vi "Evaluate Log Packet.vi"(10 "Log Packet":T1, 11 "Log Sink in":refnum<class "Log Sink.lvclass">) -> (1 "Log?":bool, 2 "Log Packet Out":T1, 3 "Log Sink out":refnum<class "Log Sink.lvclass">)   [LabVIEW 2019, in "Composed Log.lvlib" / "Log Sink.lvclass"]
uses:
  <vilib>/gpm_packages/@cs/event-logger/Source/Composed Log/Log Sink/Log Sink.lvclass
  <vilib>/gpm_packages/@cs/event-logger/Source/Composed Log/Types/Log Packet.ctl
  <vilib>/gpm_packages/@cs/event-logger/Source/Composed Log/Types/Log Level.ctl
  <vilib>/gpm_packages/@cs/event-logger/Source/Composed Log/Log Sink/Log Sink.lvclass/Log Sink.ctl
  <vilib>/gpm_packages/@cs/event-logger/Source/Composed Log/ILogFilter/ILogFilter.lvclass
  <vilib>/gpm_packages/@cs/event-logger/Source/Composed Log/Composed Log.lvlib
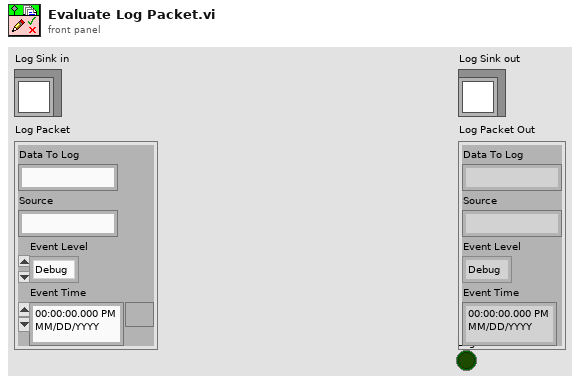
[diagram p1: front panel]
types:
  T1 = typedef "Composed Log.lvlib/Log Packet.ctl" = cluster{"Data To Log":string, "Source":string, "Event Level":T2, "Event Time":timestamp}
  T2 = typedef "Composed Log.lvlib/Log Level.ctl" = enum16{"Debug", "Info", "Warning", "Error", "Critical"}
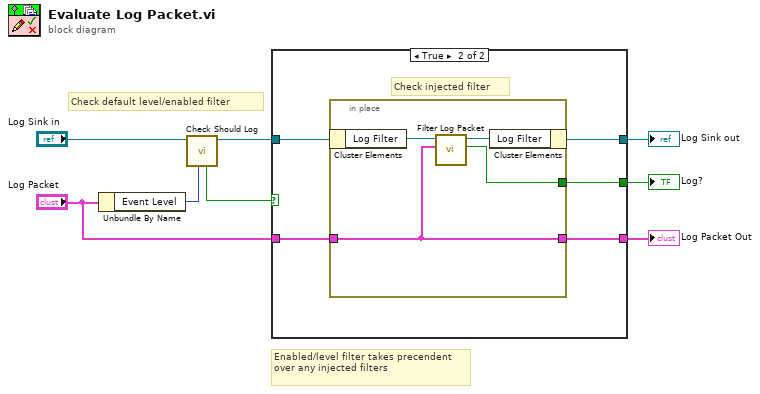
[diagram p0: block diagram]
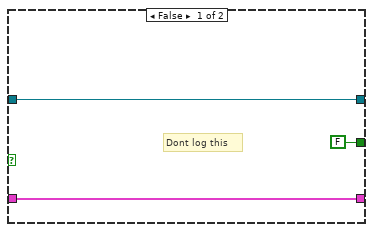
[diagram p2: hidden frame]
diagram:
  # "Enabled/level filter takes precendent over any injected filters"
  # "Check default level/enabled filter"
  n1 = Unbundle By Name("Log Packet") -> ("Event Level"=w7:T2)
  n2 = call <vilib>:"Check Should Log.vi"("LogLevel"=w7, "Log Sink in"="Log Sink in") -> ("Log Sink out"=w6:refnum<class "Log Sink.lvclass">, "Log?"=w5:bool)  [unwired: 8 in]
  n3 = case shown="True" w5 {
    tunnel: w6 -> [w11 w15]
    tunnel: "Log Packet" -> [w9 w16]
    tunnel: [w11 w14] -> w3
    tunnel: [FALSE ("Log?") w13] -> w2
    tunnel: [w9 w12] -> w1
    frame False {
      # "Dont log this"
    }
    frame True {
      # "Check injected filter"
      n4 = in-place {
        in-place-border: w16 -> [w17]
        in-place-border: [w18] -> w13
        in-place-border: [w17] -> w12
        n5 = in-place-cluster #1(w15) -> ("Log Filter"=w20:refnum<class "ILogFilter.lvclass">)
        n6 = call-dynamic "Filter Log Packet.vi"("Log Packet"=w17, "ILogFilter in"=w20) -> ("Log?"=w18:bool, "ILogFilter out"=w19:refnum<class "ILogFilter.lvclass">)  [unwired: 8 in]
        n7 = in-place-cluster #1("Log Filter"=w19) -> (w14:refnum<class "Log Sink.lvclass">)
      }
    }
  }
  "Log Sink out" <- w3
  "Log?" <- w2
  "Log Packet Out" <- w1
